vi "instantiate class.vi"(8 "error in (no error)":errorcluster, 10 "Beverage to be wrapped.lvclass":refnum<class "Beverage.lvclass">) -> (0 "error out":errorcluster, 3 "Mocha out":refnum<class "Mocha.lvclass">)   [LabVIEW 2021, in "Mocha.lvclass"]
uses:
  Mocha.lvclass
  Beverage/Beverage.lvclass
  Mocha.lvclass/Mocha.ctl
panel:
  # "Connector Pane"
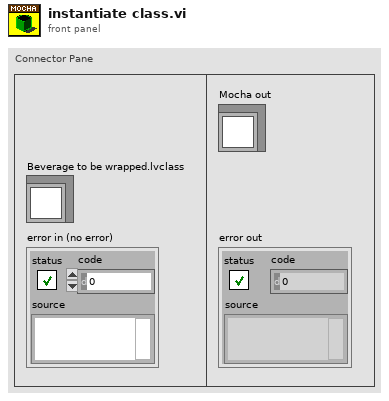
[diagram p1: front panel]
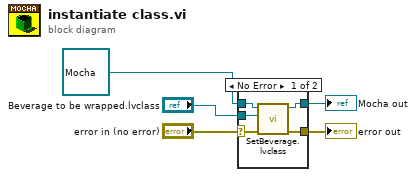
[diagram p0: block diagram]
diagram:
  n1 = case shown="No Error" "error in (no error)" {
    selector: "error in (no error)" -> [w6 w12]
    tunnel: [w9 w12] -> w5
    tunnel: [w8 w11] -> w1
    tunnel: refnum<class "Mocha.lvclass"> refnum ("Mocha in") -> [w7 w11]
    tunnel: "Beverage to be wrapped.lvclass" -> [w10 _]
    frame No Error {
      n2 = call-dynamic "SetBeverage.lvclass.vi"("error in (no error)"=w6, "Beverage.lvclass"=w10, "object in"=w7) -> ("error out"=w9:errorcluster, "object out"=w8:refnum<class "Mocha.lvclass">)  [unwired: 7 in]
    }
    frame Error {
    }
  }
  "error out" <- w5
  "Mocha out" <- w1
